vi "controle_temperatura_email.vi"() -> ()   [LabVIEW 2018]
uses:
  <vilib>/smtpClient/Set Message Text.vi
  <vilib>/smtpClient/LabVIEWSMTPClient.lvlib
panel:
  in  "Slide 2":dbl(slide) scale=0.0..35.0
  in  "Dial":dbl(knob) scale=0.0..50.0
  out "Slide":dbl(slide) scale=0.0..50.0
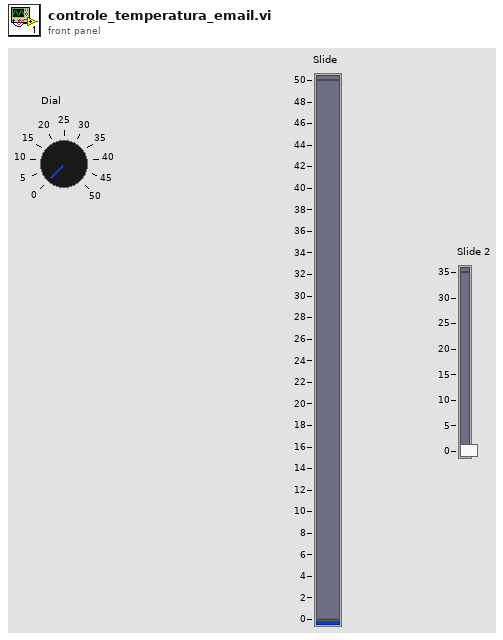
[diagram p1: front panel]
types:
  T1 = typedef "LabVIEWSMTPClient.lvlib/SmtpClientHandle.ctl" = refnum<k1>
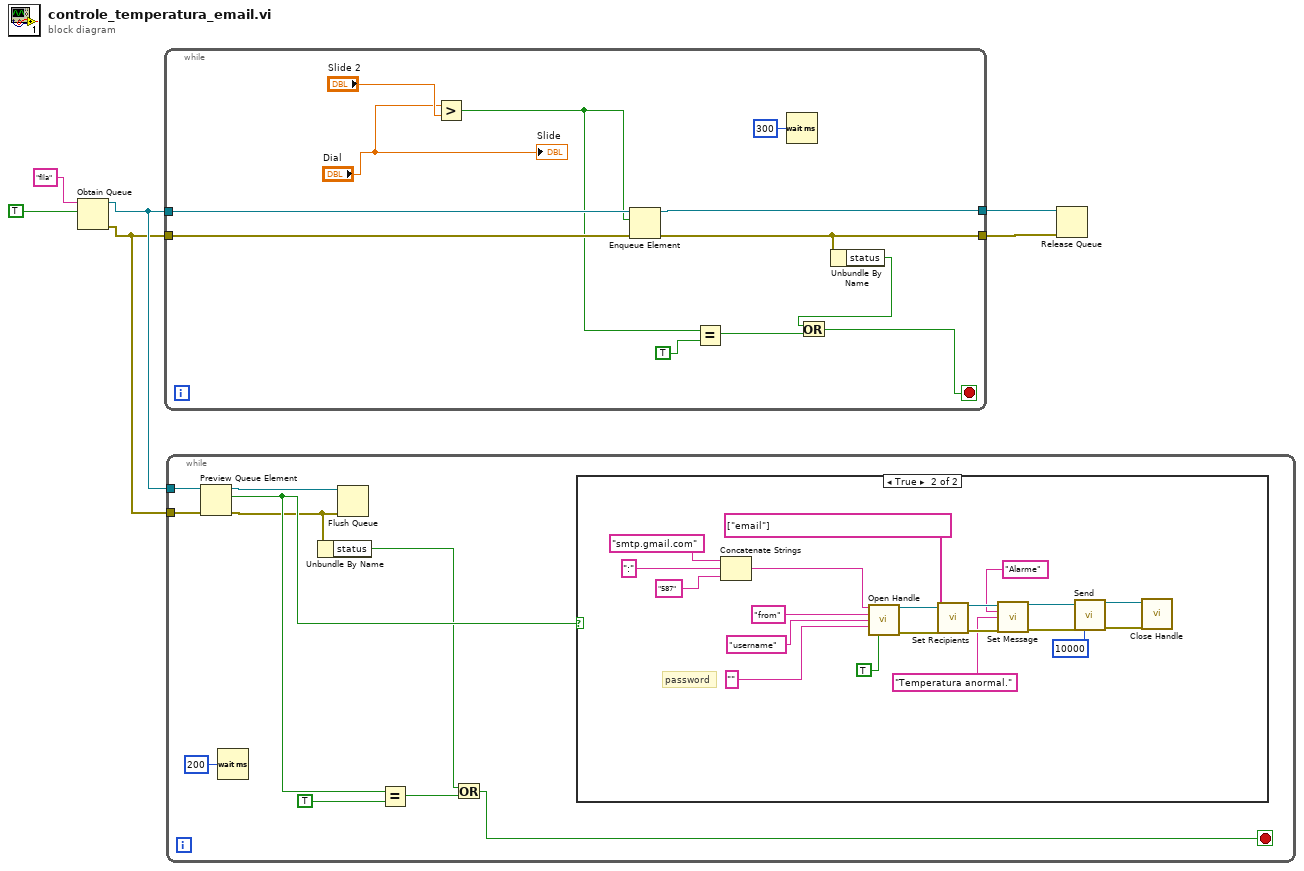
[diagram p0: block diagram]
diagram:
  n1 = Obtain Queue(name (unnamed)="fila", element data type=TRUE) -> (queue out=w2:refnum<queue>, error out=w1:errorcluster)  [unwired: 3 in, 1 out]
  n2 = while {
    tunnel: w2 -> [w18]
    tunnel: w1 -> [w17]
    tunnel: [w16] -> w4
    tunnel: [w9] -> w3
    stop <- w7 stop-if-true
    n3 = Greater?(x="Dial", y="Slide 2") -> (0:w12:bool)
    n4 = Enqueue Element(queue=w18, element=w12, error in (no error)=w17) -> (queue out=w16:refnum<queue>, error out=w9:errorcluster)  [unwired: 1 in, 1 out]
    n5 = Equal?(x=w12, y=TRUE) -> (x = y?=w10:bool)
    n6 = Wait (ms)(milliseconds to wait=u32 300) -> ()  [unwired: 1 out]
    n7 = Unbundle By Name(w9) -> ("status"=w8:bool)
    n8 = Or(x=w8, y=w10) -> (x .or. y?=w7:bool)
    "Slide" <- "Dial"
  }
  n9 = while {
    tunnel: w2 -> [w28]
    tunnel: w1 -> [w27]
    stop <- w19 stop-if-true
    n10 = Preview Queue Element(queue=w28, error in (no error)=w27) -> (queue out=w26:refnum<queue>, element=w24:bool, error out=w22:errorcluster)  [unwired: 1 in, 1 out]
    n11 = Wait (ms)(milliseconds to wait=u32 200) -> ()  [unwired: 1 out]
    n12 = Unbundle By Name(w22) -> ("status"=w21:bool)
    n13 = Flush Queue(queue=w26, error in (no error)=w22) -> ()  [unwired: 3 out]
    n14 = Equal?(x=w24, y=TRUE) -> (x = y?=w20:bool)
    n15 = Or(x=w21, y=w20) -> (x .or. y?=w19:bool)
    n16 = case shown="True" w24 {
      frame False {
      }
      frame True {
        # "password"
        n17 = Concatenate Strings("smtp.gmail.com" ("string"), ":" ("string"), "587" ("string")) -> (w29:string)
        n18 = call <vilib>:"Open Handle.vi"("server address"=w29, "from"="from", "username"="username", "password"="", "use TLS (false)"=TRUE) -> ("handle out"=w41:T1, "error out"=w40:errorcluster)  [unwired: 9 in]
        n19 = call <vilib>:"Set Recipients.vi"("handle in"=w41, "to"=string[] ["email"], "error in (no error)"=w40) -> ("handle out"=w43:T1, "error out"=w42:errorcluster)  [unwired: 11 in]
        n20 = call-poly <vilib>:"Set Message.vi"("handle in"=w43, "subject"="Alarme", "plain text message"="Temperatura anormal.", "error in (no error)"=w42) -> ("handle out"=w45:T1, "error out"=w44:errorcluster)  [unwired: 10 in]
        n21 = call <vilib>:"Send.vi"("handle in"=w45, "error in (no error)"=w44, "timeout in ms (10000)"=10000) -> ("handle out"=w47:T1, "error out"=w46:errorcluster)  [unwired: 10 in, 1 out]
        n22 = call <vilib>:"Close Handle.vi"("handle in"=w47, "error in (no error)"=w46) -> ()  [unwired: 12 in, 2 out]
      }
    }
  }
  n23 = Release Queue(queue=w4, error in (no error)=w3) -> ()  [unwired: 1 in, 3 out]
